vi "Autonomous.vi"   [LabVIEW 2017]
doc: "This VI starts when autonomous period begins, and will automatically be terminated when it ends. You can carry out timed or sensor driven operations directly to I/O or to subsystems without needing to return to the caller."
uses:
  <vilib>/Rock Robotics/WPI/Utilities/WPI_GetSetVariantRefNum.vi
  <vilib>/Rock Robotics/Network Tables/NT Read String.vi
types:
  T1 = typedef "WPI_JoystickDevRef.ctl" = cluster{"Device":T2}
  T2 = typedef "WPI_JoystickDeviceEnum.ctl" = enum16{"USB 0", "USB 1", "USB 2", "USB 3", "USB 4", "USB 5"}
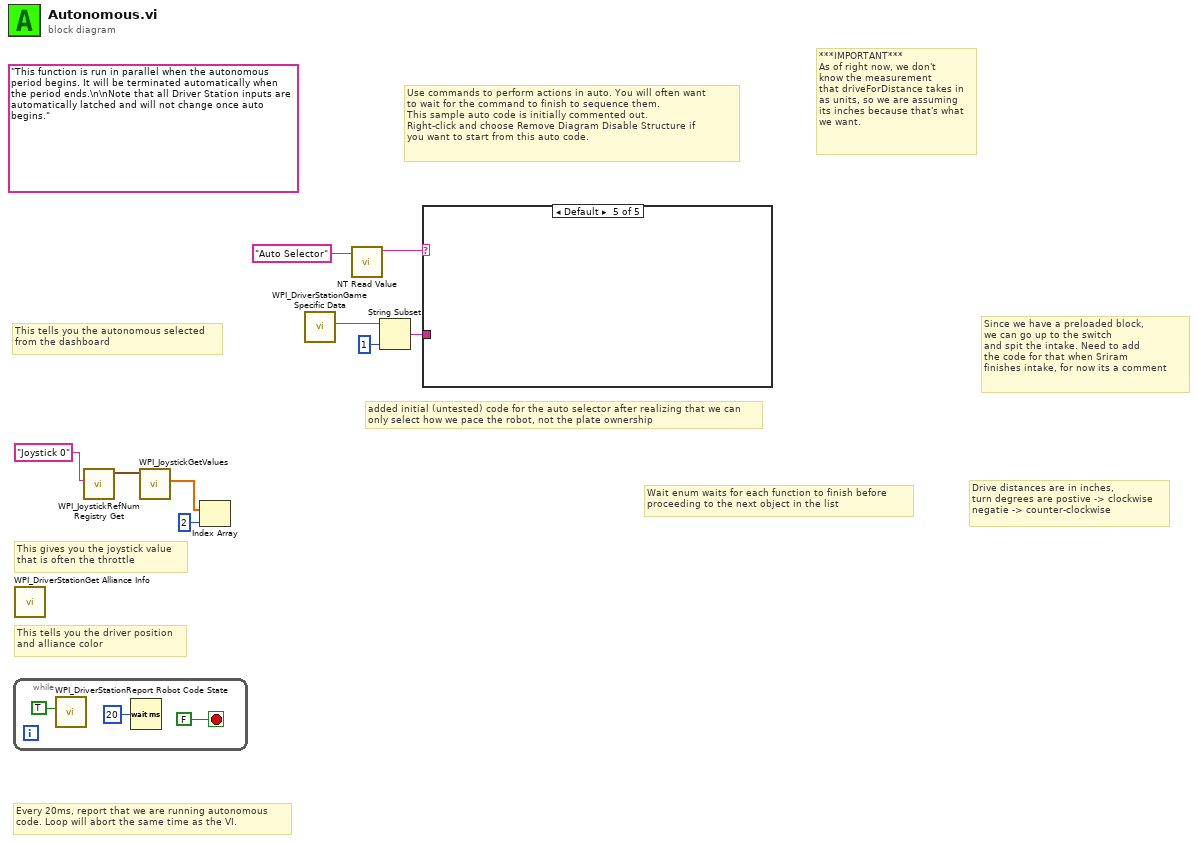
[diagram p0: block diagram]
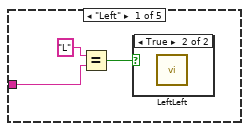
[diagram p2: hidden frame]
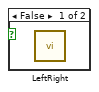
[diagram p3: hidden frame]
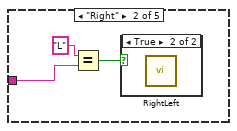
[diagram p4: hidden frame]
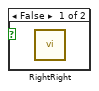
[diagram p5: hidden frame]
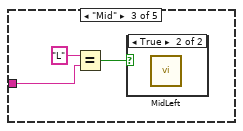
[diagram p6: hidden frame]
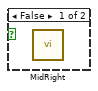
[diagram p7: hidden frame]
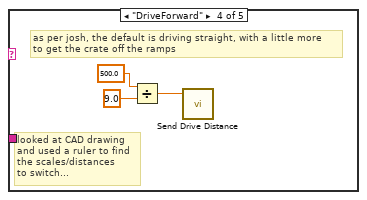
[diagram p8: hidden frame]
diagram:
  (unwired) "This function is run in parallel when the autonomous period begins. It will be terminated automatically when the period ends.\n\nNote that all Driver Station inputs are automatically latched and will not change once auto begins."
  # "added initial (untested) code for the auto selector after realizing that we can\nonly select how we pace the robot, not the plate ownership"
  # "Drive distances are in inches, \nturn degrees are postive -> clockwise\nnegatie -> counter-clockwise"
  # "Since we have a preloaded block,\nwe can go up to the switch\nand spit the intake. Need to add\nthe code for that when Sriram\nfinishes intake, for now its a comment"
  # "***IMPORTANT***\nAs of right now, we don't\nknow the measurement\nthat driveForDistance takes in\nas units, so we are assuming \nits inches because that's what\nwe want."
  # "Wait enum waits for each function to finish before\nproceeding to the next object in the list"
  # "This tells you the autonomous selected\nfrom the dashboard"
  # "Every 20ms, report that we are running autonomous\ncode. Loop will abort the same time as the VI."
  # "This gives you the joystick value\nthat is often the throttle"
  # "Use commands to perform actions in auto. You will often want\nto wait for the command to finish to sequence them.\nThis sample auto code is initially commented out. \nRight-click and choose Remove Diagram Disable Structure if\nyou want to start from this auto code."
  # "This tells you the driver position\nand alliance color"
  n1 = while {
    stop <- FALSE stop-if-true
    n2 = call <vilib>:"WPI_DriverStationReport Robot Code State.vi"("Autonomous"=TRUE) -> ()  [unwired: 10 in, 1 out]
    n3 = Wait (ms)(milliseconds to wait=u32 20) -> ()  [unwired: 1 out]
  }
  n4 = call <vilib>:"WPI_DriverStationGet Alliance Info.vi"() -> ()  [unwired: 12 out]
  n5 = call <vilib>:"WPI_JoystickRefNum Registry Get.vi"("refnum name"="Joystick 0") -> ("JoystickDevRef"=w8:T1)  [unwired: 1 in, 9 out]
  n6 = call <vilib>:"WPI_JoystickGetValues.vi"("JoystickDevRef"=w8) -> ("Axes"=w7:dbl[])  [unwired: 6 in, 4 out]
  n7 = Index Array(array=w7, index=2) -> ()  [unwired: 1 out]
  n8 = call <vilib>:"WPI_DriverStationGame Specific Data.vi"() -> ("Game Specific Data"=w4:string)  [unwired: 11 in]
  n9 = call-poly <vilib>:"NT Read Value.vi"("Name"="Auto Selector") -> ("String"=w1:string)  [unwired: 9 in, 1 out]
  n10 = String Subset(string=w4, length (rest)=1 ("length (rest)")) -> (substring=w2:string)  [unwired: 1 in]
  n11 = case shown="Default" w1 {
    tunnel: w2 -> [w13 w16 w19 _ _]
    frame "Left" {
      n12 = Equal?(x="L", y=w13) -> (x = y?=w14:bool)
      n13 = case shown="True" w14 {
        frame False {
          n14 = call "LeftRight.vi"() -> ()  [unwired: 12 in]
        }
        frame True {
          n15 = call "LeftLeft.vi"() -> ()  [unwired: 12 in]
        }
      }
    }
    frame "Right" {
      n16 = Equal?(x="L", y=w16) -> (x = y?=w17:bool)
      n17 = case shown="True" w17 {
        frame False {
          n18 = call "RightRight.vi"() -> ()  [unwired: 12 in]
        }
        frame True {
          n19 = call "RightLeft.vi"() -> ()  [unwired: 12 in]
        }
      }
    }
    frame "Mid" {
      n20 = Equal?(x="L", y=w19) -> (x = y?=w20:bool)
      n21 = case shown="True" w20 {
        frame False {
          n22 = call "MidRight.vi"() -> ()  [unwired: 12 in]
        }
        frame True {
          n23 = call "MidLeft.vi"() -> ()  [unwired: 12 in]
        }
      }
    }
    frame "DriveForward" {
      # "looked at CAD drawing\nand used a ruler to find\nthe scales/distances\nto switch..."
      # "as per josh, the default is driving straight, with a little more \nto get the crate off the ramps"
      n24 = Divide(x=500.0, y=9.0) -> (x/y=w24:dbl)
      n25 = call "Send Drive Distance.vi"("Target Distance"=w24) -> ()  [unwired: 9 in, 2 out]
    }
    frame Default {
    }
  }
